vi "Temperature Limit.vi"() -> ()   [LabVIEW 2012]
doc: "This VI simulates the acquisition of temperature, graphs the temperature, and notifies the user if the temperature is over the limit."
panel:
  in  "Start":bool
  in  "Delta t (ms)":i32(slide)=400 scale=50.0..500.0
  in  "Stop":bool
  in  "High Limit":dbl=28.0 format="%.2f"
  out "Temperature":cluster{"Temperature":dbl, "High Limit":dbl}(graph)={"Temperature"=85.88749999999999, "High Limit"=80.0}
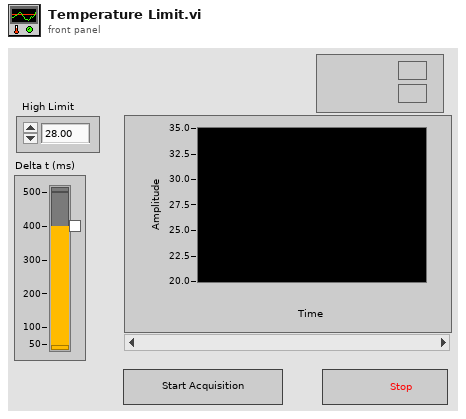
[diagram p1: front panel]
types:
  T1 = enum8{"Enabled", "Disabled", "Disabled and Grayed Out"}
  T2 = cluster{"Temperature Value":dbl, "High Limit":dbl}
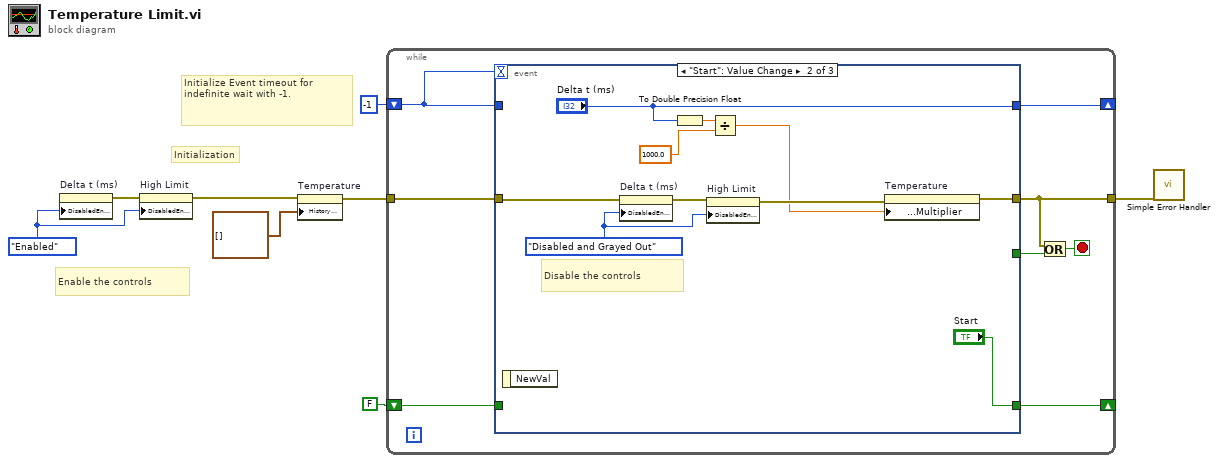
[diagram p0: block diagram]
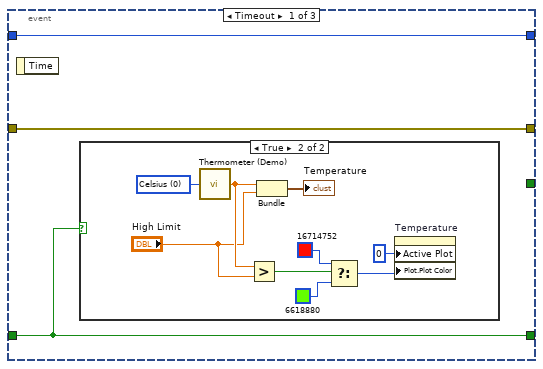
[diagram p2: hidden frame]
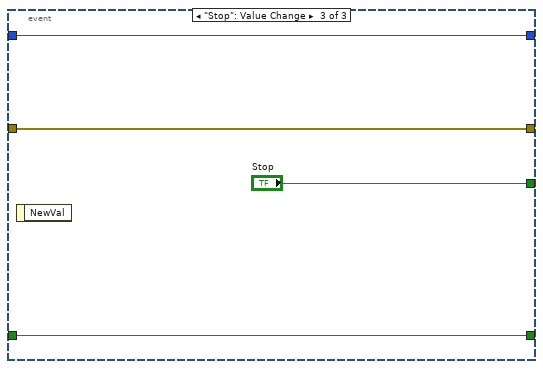
[diagram p4: hidden frame]
diagram:
  w6 = T1."Enabled" ("Disabled")
  # "Initialize Event timeout for indefinite wait with -1."
  # "Enable the controls"
  # "Initialization"
  n1 = property on="Delta t (ms)" class="Slide (strict)"("DisabledEnum"=w6) -> (error out=w5:errorcluster)  [unwired: 2 in, 1 out]
  n2 = property on="High Limit" class="DigNum (strict)"(error in=w5, "DisabledEnum"=w6) -> (error out=w4:errorcluster)  [unwired: 1 in, 1 out]
  n3 = property on="Temperature" class="WFChart (strict)"(error in=w4, "History Data"=cluster{"Temperature":dbl, "High Limit":dbl}[] []) -> (error out=w7:errorcluster)  [unwired: 1 in, 1 out]
  n4 = while {
    tunnel: w7 -> [w16]
    tunnel: [w14] -> w2
    shift-right: [w12] -> _
    shift-left: FALSE ("Start") -> [w11]
    shift-right: [w10] -> _
    shift-left: -1 ("Delta t (ms)") -> [w9]
    stop <- w15 stop-if-true
    n5 = event shown="[1] \"Start\": Value Change" {
      selector: _ -> [_ _ _]
      dyn-events: _ -> [_ _ _]
      timeout: w9 -> [_ _ _]
      tunnel: [_ _ "Stop"] -> w13
      tunnel: w16 -> [w19 w36 w41]
      tunnel: [w19 w34 w41] -> w14
      tunnel: [w17 "Start" w40] -> w12
      tunnel: w11 -> [w17 _ w40]
      tunnel: [w18 "Delta t (ms)" w39] -> w10
      tunnel: w9 -> [w18 _ w39]
      event Timeout {
        n6 = event-data() -> ()  [unwired: 1 in, 1 out]
        n7 = case shown="True" w17 {
          frame False {
          }
          frame True {
            w27 = u16 0 items=["Celsius", "Fahrenheit"] ("Units (0: Celsius)")
            n8 = call "Thermometer (Demo).vi"("Units (0: Celsius)"=w27) -> ("Temperature Value"=w26:dbl)
            n9 = Greater?(x=w26, y="High Limit") -> (0:w24:bool)
            n10 = Bundle("Temperature Value"=w26, "High Limit"="High Limit") -> (→"Temperature":T2)  [unwired: 1 in]
            n11 = Select(t=u32 16714752, s=w24, f=u32 6618880) -> (s? t:f=w23:u32)
            n12 = property on="Temperature" class="WFChart (strict)"("Active Plot"=u32 0, "Plot.Plot Color"=w23) -> ()  [unwired: 2 in, 2 out]
          }
        }
      }
      event "Start": Value Change {
        w37 = T1."Disabled and Grayed Out" ("Disabled")
        # "Disable the controls"
        n13 = event-data() -> ()  [unwired: 1 in, 1 out]
        n14 = property on="Delta t (ms)" class="Slide (strict)"(error in=w36, "DisabledEnum"=w37) -> (error out=w38:errorcluster)  [unwired: 1 in, 1 out]
        n15 = To Double Precision Float(number="Delta t (ms)") -> (double precision float=w33:dbl)
        n16 = property on="High Limit" class="DigNum (strict)"(error in=w38, "DisabledEnum"=w37) -> (error out=w35:errorcluster)  [unwired: 1 in, 1 out]
        n17 = Divide(x=w33, y=1000.0) -> (x/y=w31:dbl)
        n18 = property on="Temperature" class="WFChart (strict)"(error in=w35, "X Scale.Offset and Multiplier:Multiplier"=w31) -> (error out=w34:errorcluster)  [unwired: 1 in, 1 out]
      }
      event "Stop": Value Change {
        n19 = event-data() -> ()  [unwired: 1 in, 1 out]
      }
    }
    n20 = Or(x=w14, y=w13) -> (x .or. y?=w15:bool)
  }
  n21 = call <vilib>:"Simple Error Handler.vi"("error in (no error)"=w2) -> ()  [unwired: 4 in, 5 out]
